vi "Finish.vi"   [LabVIEW 2012]
doc: "This VI is called just before exiting. It is expected to close I/O refnum, save collected data, etc."
uses:
  <vilib>/Rock Robotics/WPI/Compressor/WPI_CompressorGetSetRefNum.vi
  <vilib>/Rock Robotics/WPI/Joystick/WPI_JoystickGetSetRefNum.vi
  <vilib>/Rock Robotics/WPI/RobotDrive/WPI_RobotDriveGetSetRefNum.vi
types:
  T1 = typedef "WPI_DigitalInputDevRef.ctl" = cluster{"DevStatus":errorcluster, "DIO Channel":T2, "Digital Module":T3}
  T2 = typedef "FPGA_DIOChannel.ctl" = enum8{"DIO 1", "DIO 2", "DIO 3", "DIO 4", "DIO 5", "DIO 6", "DIO 7", "DIO 8", "DIO 9", "DIO 10", "DIO 11", "DIO 12", "DIO 13", "DIO 14", "Invalid"}
  T3 = typedef "FPGA_TypedefDigitalModule.ctl" = enum16{"Digital Module 1", "Digital Module 2"}
  T4 = typedef "WPI_MotorControlDeviceRef.ctl" = cluster{"DeviceStatus":errorcluster, "Type":enum16{"PWM", "CAN"}, "PWM":cluster{"Digital Module":T3, "PWM Channel":T5, "DeadBand":T6}, "CAN":cluster{"Device Number":u8, "Control Mode":T7, "Semaphore":T8, "Max Vout":dbl}, "Invert":bool, "TransformRef":T9, "InvTransformRef":T9}
  T5 = typedef "FPGA_DIOPWMChannel.ctl" = enum8{"PWM 1", "PWM 2", "PWM 3", "PWM 4", "PWM 5", "PWM 6", "PWM 7", "PWM 8", "PWM 9", "PWM 10", "Invalid"}
  T6 = typedef "WPI_PWMDeadband.ctl" = cluster{"Name":string, "maxPositivePwm":i32, "minPositivePwm":i32, "centerPwm":i32, "maxNegativePwm":i32, "minNegativePwm":i32, "angularRange":u16}
  T7 = typedef "WPI_CANJaguar_ControlMode.ctl" = enum8{"Percent VBus", "Current", "Speed", "Position", "Voltage"}
  T8 = typedef "Semaphore RefNum" = refnum<k1>
  T9 = typedef "WPI_PWMTransform_ConPane.ctl" = refnum<vi>
  T10 = typedef "WPI_ServoDeviceRef.ctl" = cluster{"DeviceStatus":errorcluster, "Digital Module":T3, "PWM Channel":T5, "DeadBand":T6}
  T11 = typedef "WPI_JoystickDevRef.ctl" = cluster{"Device":T12}
  T12 = typedef "WPI_JoystickDeviceEnum.ctl" = enum16{"USB 1", "USB 2", "USB 3", "USB 4", "Kinect 1", "Kinect 2"}
  T13 = typedef "WPI_RobotDriveDevRef.ctl" = cluster{"DevStatus":errorcluster, "Motors[]":T4[], "Square Inputs":bool, "Max Output":dbl, "Isochronous":bool}
  T14 = typedef "WPI_SolenoidDevRef.ctl" = cluster{"DevStatus":errorcluster, "Solenoid Module":T15, "Forward Solenoid Channel":T16, "Reverse Solenoid Channel":T16}
  T15 = typedef "FPGA_TypedefSolenoidModule.ctl" = enum16{"Solenoid Module 1", "Solenoid Module 2"}
  T16 = typedef "WPI_SolenoidChannel.ctl" = enum8{"Solenoid 1", "Solenoid 2", "Solenoid 3", "Solenoid 4", "Solenoid 5", "Solenoid 6", "Solenoid 7", "Solenoid 8", "Invalid"}
  T17 = typedef "WPI_CompressorDevRef.ctl" = cluster{"DevStatus":errorcluster, "DigitalInputDevRef":T1, "RelayDevRef":T18}
  T18 = typedef "WPI_RelayDevRef.ctl" = cluster{"DevStatus":errorcluster, "Relay Channel":T19, "Digital Module":T3, "Relay Direction":T20}
  T19 = typedef "FPGA_DIORelayChannel.ctl" = enum8{"Relay 1", "Relay 2", "Relay 3", "Relay 4", "Relay 5", "Relay 6", "Relay 7", "Relay 8", "Invalid"}
  T20 = typedef "WPI_RelayDirection.ctl" = enum16{"Both directions", "Forward only", "Reverse only"}
  T21 = typedef "WPI_EncoderDevRef.ctl" = cluster{"DevStatus":errorcluster, "EncoderIndex":T22, "CounterIndex":T23, "DistancePerCount":dbl, "Decoding Type":T24}
  T22 = typedef "FPGA_EncoderIdx.ctl" = enum8{"Enc 0", "Enc 1", "Enc 2", "Enc 3", "Invalid"}
  T23 = typedef "FPGA_CounterCtrSystemIndex.ctl" = enum8{"Ctr 0", "Ctr 1", "Ctr 2", "Ctr 3", "Ctr 4", "Ctr 5", "Ctr 6", "Ctr 7", "Invalid"}
  T24 = typedef "WPI_EncoderType.ctl" = enum16{"1x", "2x", "4x"}
  T25 = typedef "WPI_GyroDevRef.ctl" = cluster{"DevStatus":errorcluster, "Analog Module":T26, "Analog Channel":T27, "Offset":dbl, "Gain (VoltsPerDegree/Second)":dbl}
  T26 = typedef "FPGA_TypedefAnalogModule.ctl" = enum16{"Analog Module 1", "Analog Module 2"}
  T27 = typedef "FPGA_AIChannel.ctl" = enum8{"AI 1", "AI 2", "AI 3", "AI 4", "AI 5", "AI 6", "AI 7", "AI 8", "Invalid"}
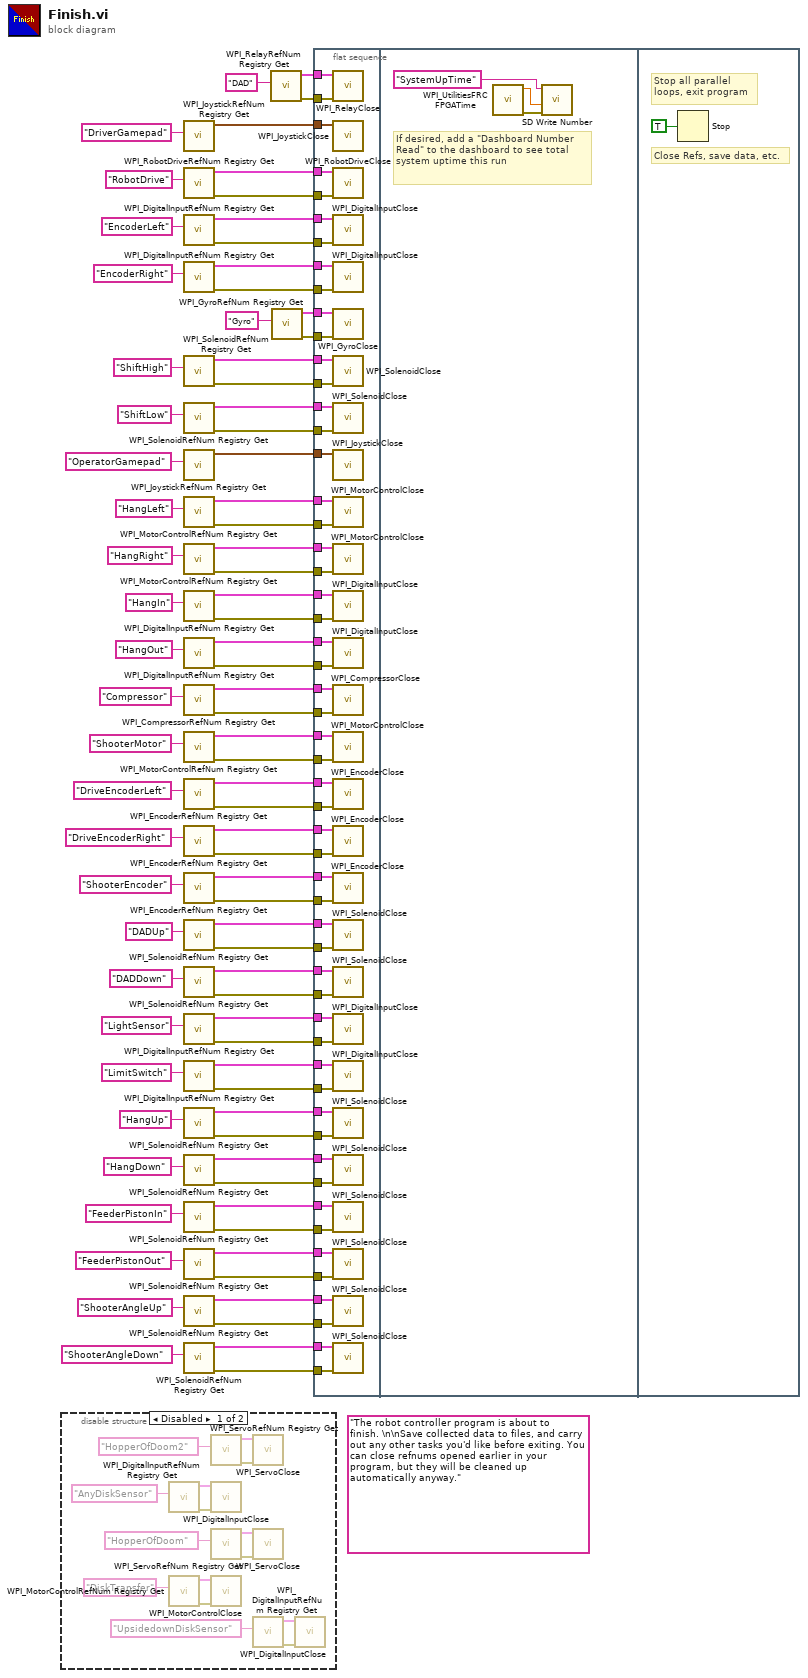
[diagram p0: block diagram]
diagram:
  (unwired) "The robot controller program is about to finish. \n\nSave collected data to files, and carry out any other tasks you'd like before exiting. You can close refnums opened earlier in your program, but they will be cleaned up automatically anyway."
  n1 = disable-structure shown="Disabled" {
    frame Disabled {
      n2 = call <vilib>:"WPI_DigitalInputRefNum Registry Get.vi"("refnum name"="AnyDiskSensor") -> ("error out"=w89:errorcluster, "DigitalInputDevRef"=w90:T1)  [unwired: 9 in]
      n3 = call <vilib>:"WPI_MotorControlRefNum Registry Get.vi"("refnum name"="DiskTransfer") -> ("error out"=w91:errorcluster, "MotorControlDevRef"=w92:T4)  [unwired: 9 in]
      n4 = call <vilib>:"WPI_ServoRefNum Registry Get.vi"("refnum name"="HopperOfDoom2") -> ("error out"=w83:errorcluster, "ServoDeviceRef"=w84:T10)  [unwired: 9 in]
      n5 = call <vilib>:"WPI_DigitalInputClose.vi"("error in (no error)"=w89, "DigitalInputDevRef"=w90) -> ()  [unwired: 9 in, 1 out]
      n6 = call <vilib>:"WPI_ServoRefNum Registry Get.vi"("refnum name"="HopperOfDoom") -> ("error out"=w85:errorcluster, "ServoDeviceRef"=w86:T10)  [unwired: 9 in]
      n7 = call <vilib>:"WPI_MotorControlClose.vi"("error in (no error)"=w91, "MotorControlDevRef"=w92) -> ()  [unwired: 9 in, 1 out]
      n8 = call <vilib>:"WPI_ServoClose.vi"("error in (no error)"=w83, "MotorControlDevRef"=w84) -> ()  [unwired: 9 in, 1 out]
      n9 = call <vilib>:"WPI_ServoClose.vi"("error in (no error)"=w85, "MotorControlDevRef"=w86) -> ()  [unwired: 9 in, 1 out]
      n10 = call <vilib>:"WPI_DigitalInputRefNum Registry Get.vi"("refnum name"="UpsidedownDiskSensor") -> ("error out"=w87:errorcluster, "DigitalInputDevRef"=w88:T1)  [unwired: 9 in]
      n11 = call <vilib>:"WPI_DigitalInputClose.vi"("error in (no error)"=w87, "DigitalInputDevRef"=w88) -> ()  [unwired: 9 in, 1 out]
    }
    frame Enabled {
    }
  }
  n12 = call <vilib>:"WPI_JoystickRefNum Registry Get.vi"("refnum name"="DriverGamepad") -> ("JoystickDevRef"=w79:T11)  [unwired: 1 in, 9 out]
  n13 = call <vilib>:"WPI_RobotDriveRefNum Registry Get.vi"("refnum name"="RobotDrive") -> ("error out"=w78:errorcluster, "RobotDriveDevRef"=w80:T13)  [unwired: 1 in, 8 out]
  n14 = call <vilib>:"WPI_DigitalInputRefNum Registry Get.vi"("refnum name"="EncoderLeft") -> ("error out"=w72:errorcluster, "DigitalInputDevRef"=w73:T1)  [unwired: 9 in]
  n15 = call <vilib>:"WPI_DigitalInputRefNum Registry Get.vi"("refnum name"="EncoderRight") -> ("error out"=w71:errorcluster, "DigitalInputDevRef"=w66:T1)  [unwired: 9 in]
  n16 = call <vilib>:"WPI_SolenoidRefNum Registry Get.vi"("refnum name"="ShiftHigh") -> ("error out"=w69:errorcluster, "SolenoidDevRef"=w70:T14)  [unwired: 9 in]
  n17 = call <vilib>:"WPI_SolenoidRefNum Registry Get.vi"("refnum name"="ShiftLow") -> ("error out"=w67:errorcluster, "SolenoidDevRef"=w68:T14)  [unwired: 9 in]
  n18 = call <vilib>:"WPI_JoystickRefNum Registry Get.vi"("refnum name"="OperatorGamepad") -> ("JoystickDevRef"=w65:T11)  [unwired: 1 in, 9 out]
  n19 = call <vilib>:"WPI_MotorControlRefNum Registry Get.vi"("refnum name"="HangLeft") -> ("error out"=w61:errorcluster, "MotorControlDevRef"=w62:T4)  [unwired: 9 in]
  n20 = call <vilib>:"WPI_MotorControlRefNum Registry Get.vi"("refnum name"="HangRight") -> ("error out"=w60:errorcluster, "MotorControlDevRef"=w59:T4)  [unwired: 9 in]
  n21 = call <vilib>:"WPI_DigitalInputRefNum Registry Get.vi"("refnum name"="HangIn") -> ("error out"=w56:errorcluster, "DigitalInputDevRef"=w57:T1)  [unwired: 9 in]
  n22 = call <vilib>:"WPI_DigitalInputRefNum Registry Get.vi"("refnum name"="HangOut") -> ("error out"=w53:errorcluster, "DigitalInputDevRef"=w52:T1)  [unwired: 9 in]
  n23 = call <vilib>:"WPI_CompressorRefNum Registry Get.vi"("refnum name"="Compressor") -> ("error out"=w49:errorcluster, "CompressorDevRef"=w50:T17)  [unwired: 9 in]
  n24 = call <vilib>:"WPI_MotorControlRefNum Registry Get.vi"("refnum name"="ShooterMotor") -> ("error out"=w48:errorcluster, "MotorControlDevRef"=w47:T4)  [unwired: 9 in]
  n25 = call <vilib>:"WPI_EncoderRefNum Registry Get.vi"("refnum name"="DriveEncoderLeft") -> ("error out"=w43:errorcluster, "EncoderDevRef"=w44:T21)  [unwired: 9 in]
  n26 = call <vilib>:"WPI_EncoderRefNum Registry Get.vi"("refnum name"="DriveEncoderRight") -> ("error out"=w42:errorcluster, "EncoderDevRef"=w41:T21)  [unwired: 9 in]
  n27 = call <vilib>:"WPI_EncoderRefNum Registry Get.vi"("refnum name"="ShooterEncoder") -> ("error out"=w37:errorcluster, "EncoderDevRef"=w38:T21)  [unwired: 9 in]
  n28 = call <vilib>:"WPI_SolenoidRefNum Registry Get.vi"("refnum name"="DADUp") -> ("error out"=w34:errorcluster, "SolenoidDevRef"=w35:T14)  [unwired: 9 in]
  n29 = call <vilib>:"WPI_SolenoidRefNum Registry Get.vi"("refnum name"="DADDown") -> ("error out"=w33:errorcluster, "SolenoidDevRef"=w32:T14)  [unwired: 9 in]
  n30 = call <vilib>:"WPI_DigitalInputRefNum Registry Get.vi"("refnum name"="LightSensor") -> ("error out"=w26:errorcluster, "DigitalInputDevRef"=w27:T1)  [unwired: 9 in]
  n31 = call <vilib>:"WPI_DigitalInputRefNum Registry Get.vi"("refnum name"="LimitSwitch") -> ("error out"=w23:errorcluster, "DigitalInputDevRef"=w22:T1)  [unwired: 9 in]
  n32 = call <vilib>:"WPI_SolenoidRefNum Registry Get.vi"("refnum name"="HangUp") -> ("error out"=w19:errorcluster, "SolenoidDevRef"=w18:T14)  [unwired: 9 in]
  n33 = call <vilib>:"WPI_SolenoidRefNum Registry Get.vi"("refnum name"="HangDown") -> ("error out"=w14:errorcluster, "SolenoidDevRef"=w15:T14)  [unwired: 9 in]
  n34 = call <vilib>:"WPI_SolenoidRefNum Registry Get.vi"("refnum name"="FeederPistonIn") -> ("error out"=w13:errorcluster, "SolenoidDevRef"=w12:T14)  [unwired: 9 in]
  n35 = call <vilib>:"WPI_SolenoidRefNum Registry Get.vi"("refnum name"="FeederPistonOut") -> ("error out"=w8:errorcluster, "SolenoidDevRef"=w9:T14)  [unwired: 9 in]
  n36 = call <vilib>:"WPI_SolenoidRefNum Registry Get.vi"("refnum name"="ShooterAngleUp") -> ("error out"=w7:errorcluster, "SolenoidDevRef"=w6:T14)  [unwired: 9 in]
  n37 = call <vilib>:"WPI_SolenoidRefNum Registry Get.vi"("refnum name"="ShooterAngleDown") -> ("error out"=w2:errorcluster, "SolenoidDevRef"=w3:T14)  [unwired: 9 in]
  n38 = call <vilib>:"WPI_RelayRefNum Registry Get.vi"("refnum name"="DAD") -> ("error out"=w28:errorcluster, "RelayDevRef"=w29:T18)  [unwired: 9 in]
  n39 = call <vilib>:"WPI_GyroRefNum Registry Get.vi"("refnum name"="Gyro") -> ("error out"=w1:errorcluster, "GyroDevRef"=w21:T25)  [unwired: 9 in]
  n40 = flat-sequence {
    tunnel: w80 -> [w151]
    tunnel: w79 -> [w150]
    tunnel: w78 -> [w149]
    tunnel: w73 -> [w148]
    tunnel: w72 -> [w147]
    tunnel: w71 -> [w146]
    tunnel: w70 -> [w145]
    tunnel: w69 -> [w144]
    tunnel: w68 -> [w143]
    tunnel: w67 -> [w142]
    tunnel: w66 -> [w141]
    tunnel: w65 -> [w140]
    tunnel: w62 -> [w139]
    tunnel: w61 -> [w138]
    tunnel: w59 -> [w136]
    tunnel: w60 -> [w137]
    tunnel: w56 -> [w134]
    tunnel: w57 -> [w135]
    tunnel: w53 -> [w133]
    tunnel: w52 -> [w132]
    tunnel: w50 -> [w131]
    tunnel: w49 -> [w130]
    tunnel: w47 -> [w128]
    tunnel: w48 -> [w129]
    tunnel: w44 -> [w127]
    tunnel: w43 -> [w126]
    tunnel: w41 -> [w124]
    tunnel: w42 -> [w125]
    tunnel: w38 -> [w123]
    tunnel: w37 -> [w122]
    tunnel: w35 -> [w121]
    tunnel: w34 -> [w120]
    tunnel: w32 -> [w118]
    tunnel: w33 -> [w119]
    tunnel: w29 -> [w117]
    tunnel: w28 -> [w116]
    tunnel: w26 -> [w114]
    tunnel: w27 -> [w115]
    tunnel: w23 -> [w113]
    tunnel: w22 -> [w112]
    tunnel: w21 -> [w111]
    tunnel: w18 -> [w109]
    tunnel: w19 -> [w110]
    tunnel: w15 -> [w108]
    tunnel: w14 -> [w107]
    tunnel: w12 -> [w105]
    tunnel: w13 -> [w106]
    tunnel: w9 -> [w104]
    tunnel: w8 -> [w103]
    tunnel: w6 -> [w101]
    tunnel: w7 -> [w102]
    tunnel: w3 -> [w100]
    tunnel: w2 -> [w99]
    tunnel: w1 -> [w98]
    frame #0 {
      n41 = call <vilib>:"WPI_RelayClose.vi"("error in (no error)"=w116, "RelayDevRef"=w117) -> ()  [unwired: 9 in, 1 out]
      n42 = call <vilib>:"WPI_JoystickClose.vi"("JoystickDevRef"=w150) -> ()  [unwired: 11 out]
      n43 = call <vilib>:"WPI_RobotDriveClose.vi"("error in (no error)"=w149, "RobotDriveDevRef"=w151) -> ()  [unwired: 10 out]
      n44 = call <vilib>:"WPI_DigitalInputClose.vi"("error in (no error)"=w147, "DigitalInputDevRef"=w148) -> ()  [unwired: 9 in, 1 out]
      n45 = call <vilib>:"WPI_DigitalInputClose.vi"("error in (no error)"=w146, "DigitalInputDevRef"=w141) -> ()  [unwired: 9 in, 1 out]
      n46 = call <vilib>:"WPI_GyroClose.vi"("error in (no error)"=w98, "GyroDevRef"=w111) -> ()  [unwired: 9 in, 1 out]
      n47 = call <vilib>:"WPI_SolenoidClose.vi"("error in (no error)"=w144, "SolenoidDevRef"=w145) -> ()  [unwired: 9 in, 1 out]
      n48 = call <vilib>:"WPI_SolenoidClose.vi"("error in (no error)"=w142, "SolenoidDevRef"=w143) -> ()  [unwired: 9 in, 1 out]
      n49 = call <vilib>:"WPI_JoystickClose.vi"("JoystickDevRef"=w140) -> ()  [unwired: 11 out]
      n50 = call <vilib>:"WPI_MotorControlClose.vi"("error in (no error)"=w138, "MotorControlDevRef"=w139) -> ()  [unwired: 9 in, 1 out]
      n51 = call <vilib>:"WPI_MotorControlClose.vi"("error in (no error)"=w137, "MotorControlDevRef"=w136) -> ()  [unwired: 9 in, 1 out]
      n52 = call <vilib>:"WPI_DigitalInputClose.vi"("error in (no error)"=w134, "DigitalInputDevRef"=w135) -> ()  [unwired: 9 in, 1 out]
      n53 = call <vilib>:"WPI_DigitalInputClose.vi"("error in (no error)"=w133, "DigitalInputDevRef"=w132) -> ()  [unwired: 9 in, 1 out]
      n54 = call <vilib>:"WPI_CompressorClose.vi"("error in (no error)"=w130, "CompressorDevRef"=w131) -> ()  [unwired: 9 in, 1 out]
      n55 = call <vilib>:"WPI_MotorControlClose.vi"("error in (no error)"=w129, "MotorControlDevRef"=w128) -> ()  [unwired: 9 in, 1 out]
      n56 = call <vilib>:"WPI_EncoderClose.vi"("error in (no error)"=w126, "EncoderDevRef"=w127) -> ()  [unwired: 9 in, 1 out]
      n57 = call <vilib>:"WPI_EncoderClose.vi"("error in (no error)"=w125, "EncoderDevRef"=w124) -> ()  [unwired: 9 in, 1 out]
      n58 = call <vilib>:"WPI_EncoderClose.vi"("error in (no error)"=w122, "EncoderDevRef"=w123) -> ()  [unwired: 9 in, 1 out]
      n59 = call <vilib>:"WPI_SolenoidClose.vi"("error in (no error)"=w120, "SolenoidDevRef"=w121) -> ()  [unwired: 9 in, 1 out]
      n60 = call <vilib>:"WPI_SolenoidClose.vi"("error in (no error)"=w119, "SolenoidDevRef"=w118) -> ()  [unwired: 9 in, 1 out]
      n61 = call <vilib>:"WPI_DigitalInputClose.vi"("error in (no error)"=w114, "DigitalInputDevRef"=w115) -> ()  [unwired: 9 in, 1 out]
      n62 = call <vilib>:"WPI_DigitalInputClose.vi"("error in (no error)"=w113, "DigitalInputDevRef"=w112) -> ()  [unwired: 9 in, 1 out]
      n63 = call <vilib>:"WPI_SolenoidClose.vi"("error in (no error)"=w110, "SolenoidDevRef"=w109) -> ()  [unwired: 9 in, 1 out]
      n64 = call <vilib>:"WPI_SolenoidClose.vi"("error in (no error)"=w107, "SolenoidDevRef"=w108) -> ()  [unwired: 9 in, 1 out]
      n65 = call <vilib>:"WPI_SolenoidClose.vi"("error in (no error)"=w106, "SolenoidDevRef"=w105) -> ()  [unwired: 9 in, 1 out]
      n66 = call <vilib>:"WPI_SolenoidClose.vi"("error in (no error)"=w103, "SolenoidDevRef"=w104) -> ()  [unwired: 9 in, 1 out]
      n67 = call <vilib>:"WPI_SolenoidClose.vi"("error in (no error)"=w102, "SolenoidDevRef"=w101) -> ()  [unwired: 9 in, 1 out]
      n68 = call <vilib>:"WPI_SolenoidClose.vi"("error in (no error)"=w99, "SolenoidDevRef"=w100) -> ()  [unwired: 9 in, 1 out]
    }
    frame #1 {
      # "If desired, add a \"Dashboard Number Read\" to the dashboard to see total system uptime this run"
      n69 = call <vilib>:"WPI_UtilitiesFRC FPGATime.vi"() -> ("error out"=w154:errorcluster, "FPGA Time"=w153:dbl)  [unwired: 10 in]
      n70 = call <vilib>:"SD Write Number.vi"("error in"=w154, "Numeric"=w153, "Name"="SystemUpTime") -> ()  [unwired: 7 in, 2 out]
    }
    frame #2 {
      # "Close Refs, save data, etc."
      # "Stop all parallel\nloops, exit program"
      n71 = Stop(stop? (T)=TRUE ("Quit")) -> ()
    }
  }
